vi "Msg - FP Elt - (N) En-Dis.vi"(0 "Messages":T1[](array[typedef]), 11 "error in (no error)":errorcluster) -> (15 "error out":errorcluster)   [LabVIEW 2016, in "Error Handler - Logger.lvlib"]
doc: "Send (N) Messages to this Module to enable and/or disable certain of its FP Elements."
uses:
  Error Handler - Logger.lvlib
  Controls/FP - Enable_Disable.ctl
  Controls/FP - Actionable Element.ctl
  Controls/Message.ctl
  Controls/Module - States.ctl
  Modules.ctl
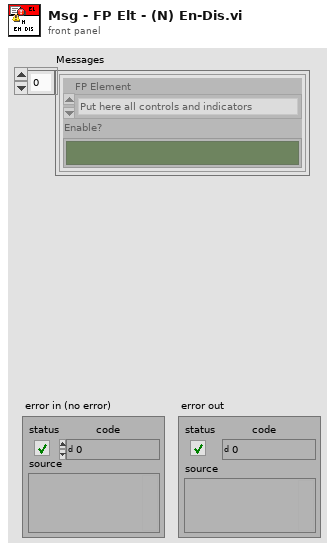
[diagram p1: front panel]
types:
  T1 = typedef "Error Handler - Logger.lvlib/FP - Enable_Disable.ctl" = cluster{"FP Element":T2, "Enable?":bool}
  T2 = typedef "Error Handler - Logger.lvlib/FP - Actionable Element.ctl" = enum16{"Put here all controls and indicators", "belonging to the UI of this module", "whose value can ", "be updated programatically", "or which can be enabled or disabled", ""}
  T3 = typedef "Error Handler - Logger.lvlib/Message.ctl" = cluster{"State":T4, "Data":variant, "Originating Module":T5}
  T4 = typedef "Error Handler - Logger.lvlib/Module - States.ctl" = enum16{"Initialize", "Event ", "Send data", "FP Element: Update", "FP Element: Disable/Enable", "Timer: Setup", "Terminate", "--------Template----------", "Process Error", "Log ", "Log Error"}
  T5 = typedef "Error Handler - Logger.lvlib/Modules.ctl" = enum16{"Controller", "Error Handler - Logger"}
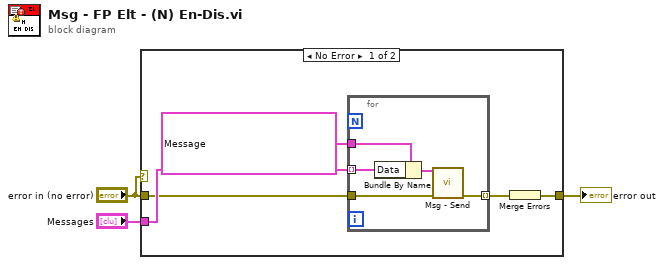
[diagram p0: block diagram]
diagram:
  n1 = case shown="No Error" "error in (no error)" {
    tunnel: [w4 w14] -> w3
    tunnel: "error in (no error)" -> [w6 w14]
    tunnel: "Messages" -> [w8 _]
    frame No Error {
      n2 = for {
        tunnel: w8 -> [w13] mode=indexing
        tunnel: T3 {"State"=enum."FP Element: Disable/Enable", "Data"=variant, "Originating Module"=enum."Controller"} ("Message") -> [w12]
        tunnel: w6 -> [w10]
        tunnel: [w9] -> w5 mode=indexing
        n3 = Bundle By Name(cluster=w12, "Data"=w13) -> (w11:T3)
        n4 = call "Msg - Send.vi"("Message"=w11, "error in (no error)"=w10) -> ("error out"=w9:errorcluster)  [unwired: 13 in]
      }
      n5 = Merge Errors(w5) -> (w4:errorcluster)
    }
    frame Error {
    }
  }
  "error out" <- w3
